vi "FROG_IFFT.vi"(5 "Overlayed Complex Electric Field":cdb[][](array[numeric])) -> (2 "Traced Pulse":cdb[][](array[numeric]))   [LabVIEW 2013]
uses:
  <vilib>/Analysis/2dsp.llb/Inverse Complex FFT.vi
  <vilib>/Analysis/NI_AALPro.lvlib
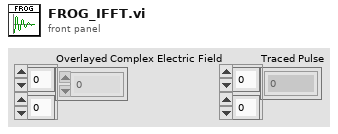
[diagram p1: front panel]
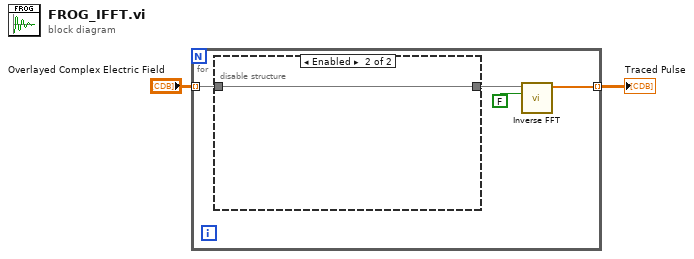
[diagram p0: block diagram]
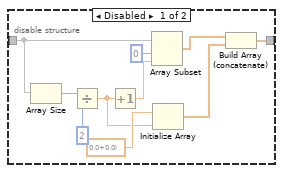
[diagram p2: hidden frame]
diagram:
  n1 = for {
    tunnel: "Overlayed Complex Electric Field" -> [w4] mode=indexing
    tunnel: [w6] -> w2 mode=indexing
    n2 = disable-structure shown="Enabled" {
      disable-tunnel: w4 -> [w16 w17]
      disable-tunnel: [w11 w17] -> w3
      frame Disabled {
        n3 = Array Size(array=w16) -> (size(s)=w15:i32)
        n4 = Divide(x=w15, y=2) -> (x/y=w8:dbl)
        n5 = Increment(x=w8) -> (x+1=w7:dbl)
        n6 = Array Subset(array=w16, index=0, length=w7) -> (w13:cdb[])
        n7 = Initialize Array(cdb 0.0+0.0i, w8) -> (w12:cdb[])
        n8 = Build Array (concatenate)(w13, w12) -> (w11:cdb[])
      }
      frame Enabled {
      }
    }
    n9 = call-poly <vilib>:"Inverse FFT.vi"("shift?"=FALSE, "FFT {X}"=w3) -> ("X"=w6:cdb[])  [unwired: 8 in, 1 out]
  }
  "Traced Pulse" <- w2
